vi "Dispose_.vi"(8 "error in (no error)":errorcluster, 11 "BombedWall":refnum<class "BombedWall.lvclass">) -> (0 "error out":errorcluster)   [LabVIEW 2020]
uses:
  BombedWall.lvclass
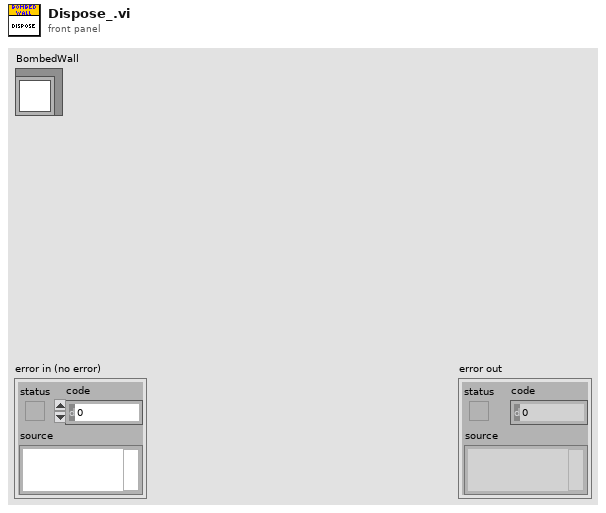
[diagram p1: front panel]
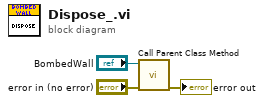
[diagram p0: block diagram]
diagram:
  n1 = call-parent "Call Parent Class Method"("error in (no error)"="error in (no error)", "Wall"="BombedWall") -> ("error out"=→"error out":errorcluster)  [unwired: 9 in]
